vi "RP100.IDN.vi"(8 "error in (no error)":errorcluster, 11 "VISA resource name":refnum<visa-resource-name>) -> (0 "error out":errorcluster, 2 "*IDN?":string, 3 "VISA Refnum out":refnum<visa-resource-name>)   [LabVIEW 2019, in "Inst.RP100.lvclass"]
uses:
  Inst.RP100.lvclass
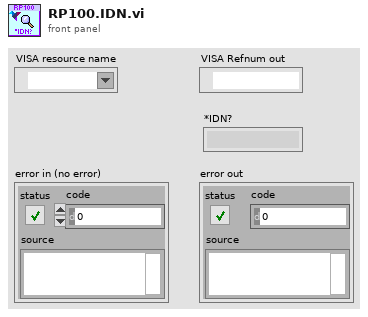
[diagram p1: front panel]
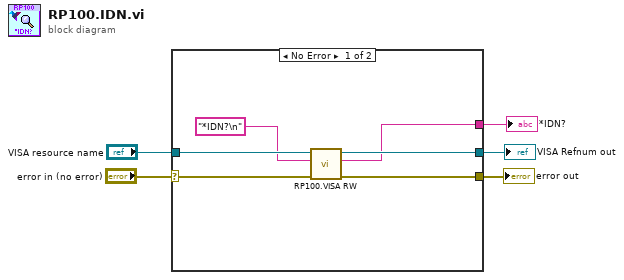
[diagram p0: block diagram]
diagram:
  n1 = case shown="No Error" "error in (no error)" {
    selector: "error in (no error)" -> [w8 w13]
    tunnel: [w11 w12] -> w5
    tunnel: "VISA resource name" -> [w10 w12]
    tunnel: [w9 w13] -> w3
    tunnel: [w7 _] -> w2
    frame No Error {
      n2 = call "RP100.VISA RW.vi"("error in (no error)"=w8, "Write"="*IDN?\n" ("format string"), "VISA Refnum in"=w10) -> ("error out"=w9:errorcluster, "Read"=w7:string, "VISA Refnum out"=w11:refnum<visa-resource-name>)  [unwired: 6 in]
    }
    frame Error {
    }
  }
  "*IDN?" <- w2
  "VISA Refnum out" <- w5
  "error out" <- w3
